vi "Camera.vi"() -> ()   [LabVIEW 2013]
uses:
  Global.vi
panel:
  in  "stop":bool
  in  "Tab Control":enum32{"Camera", "Settings"}(tab)=enum."Settings"
  in  "Pause":bool
  out "Image":T1(plugin-control)
  in  "Zoom":bool
  out "image":i32=1
  in  "max":i32=35000
  in  "min":i32=-35000
  out "Saving":bool=TRUE
  in  "Exposure (ms)":i32=1000
  in  "Colour":u32(ring) items=["Grayscale", "Binary", "Gradient", "Rainbow", "Temperature", "User Defined"]
  out "Image Pixels (I16)":i16[][](array[numeric])=[[-16415, 18069, 30328, 20956, -23719, 10482, 28186, -29010], [32361, 12219, 10367, -21635, -896, 25505, 19841, -22848], [6729, -31829, 19463, -4149, -20618, -4209, 13041, -16224], [-17471, 350, -7557, -30697, 2278, 13038, -13103, -35], [3415, -32273, -5585, -1036, 17798, -25055, 1491, 1884], [10011, -30652, 18549, 30390, 28432, 1602, 13207, 32079], [-19764, -14787, -1537, 876, -26796, 32102, -30010, 10632], [24360, 23280, -15147, -24738, 4016, -28871, -32567, -30048]]
  out "error out":errorcluster
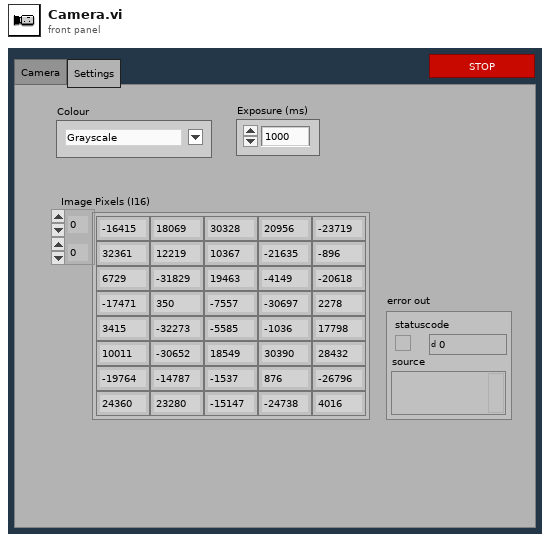
[diagram p1: front panel]
types:
  T1 = typedef "IMAQ Image.ctl" = refnum<image>
  T2 = typedef "Image Type" = u32
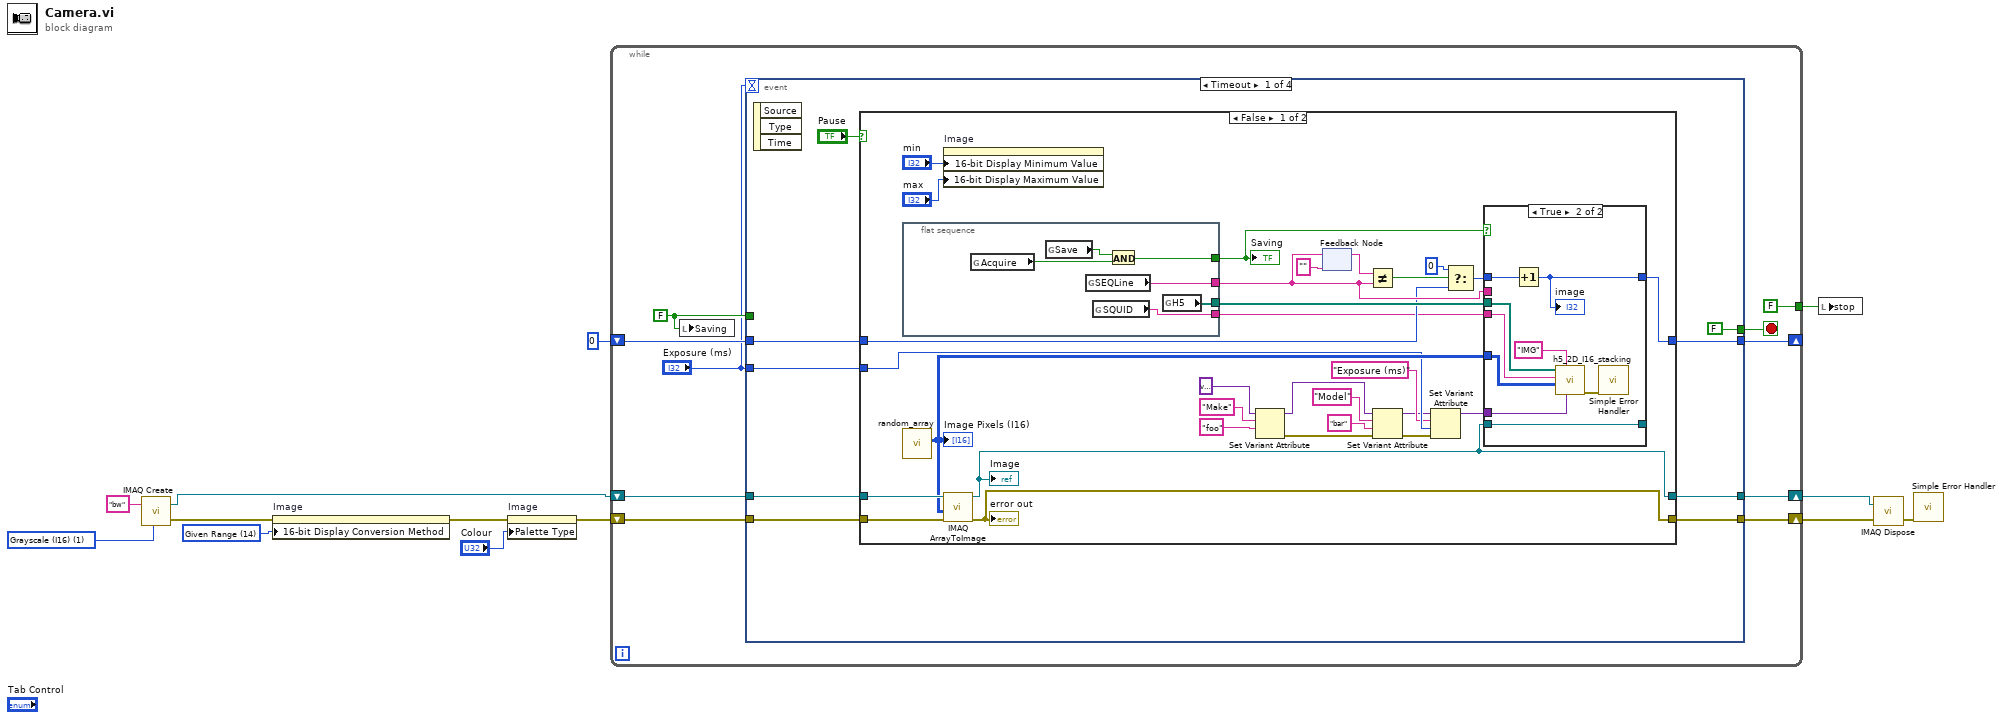
[diagram p0: block diagram]
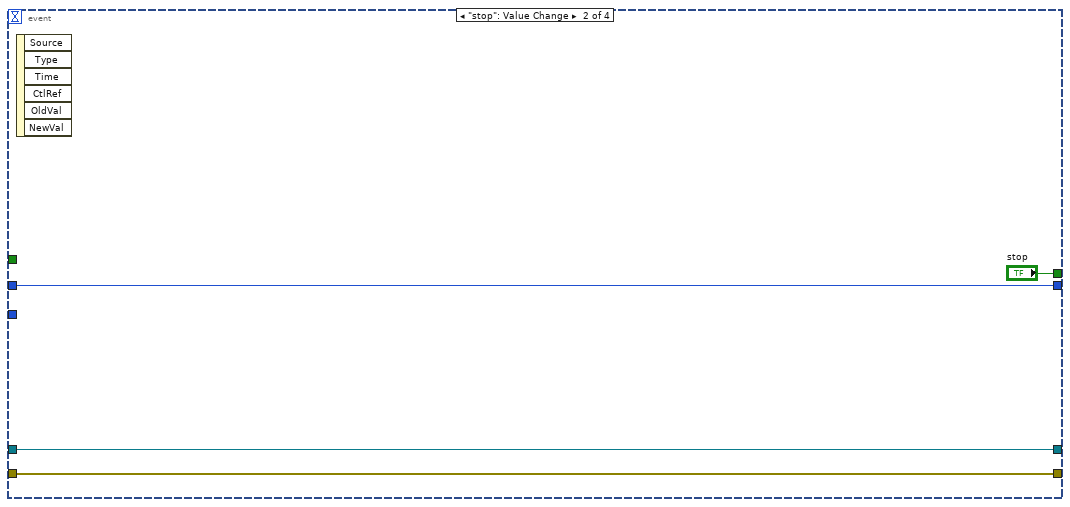
[diagram p4: hidden frame]
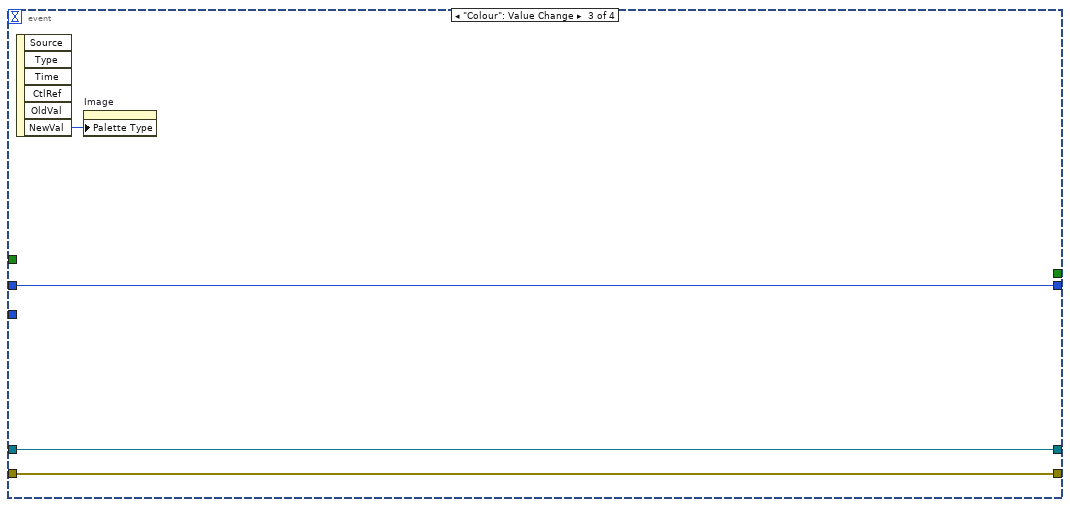
[diagram p5: hidden frame]
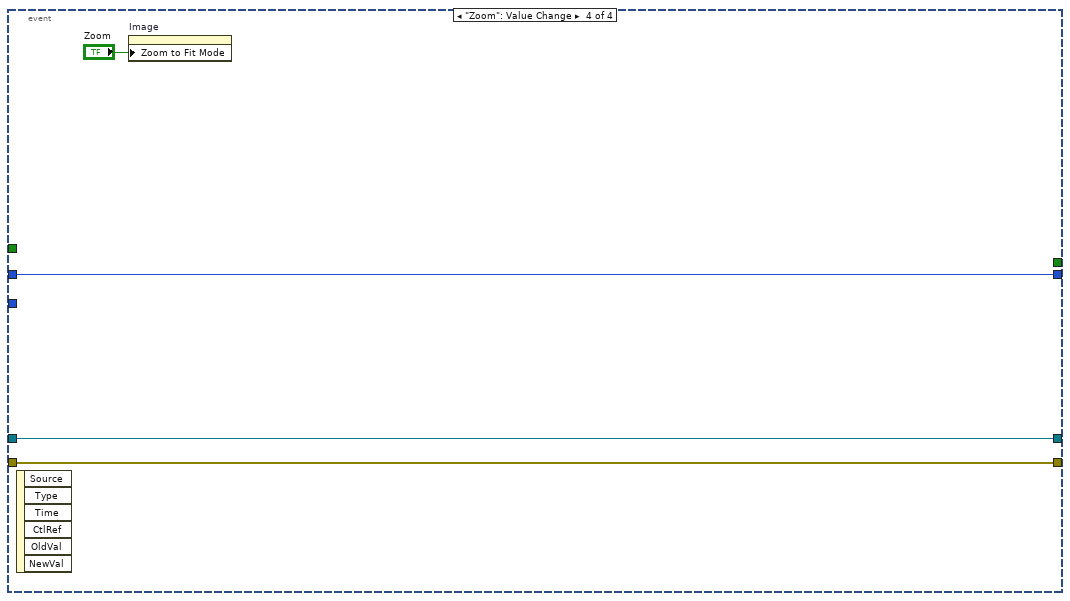
[diagram p6: hidden frame]
diagram:
  w11 = u32 14 items=["Default"=10, "Most Significant Bits"=11, "Full Dynamic"=12, "Downshift"=13, "Given Range"=14, "90% Dynamic"=15, "Given Percent Range"=16] ("16-bit Display Mapping:Conversion Method")
  w13 = T2 1 items=["Grayscale (U8)", "Grayscale (I16)", "Grayscale (SGL)", "Complex (CSG)", "RGB (U32)", "HSL (U32)", "RGB (U64)", "Grayscale (U16)"] ("Image Type")
  n1 = call "IMAQ Create"("Image Name"="bw", "Image Type"=w13) -> ("New Image"=w4:T1, "error out"=w3:errorcluster)  [unwired: 3 in]
  n2 = property on="Image" class="ImageControl"(error in=w3, "16-bit Display Conversion Method"=w11) -> (error out=w8:errorcluster)  [unwired: 1 in, 1 out]
  n3 = property on="Image" class="ImageControl"(error in=w8, "Palette Type"="Colour") -> (error out=w2:errorcluster)  [unwired: 1 in, 1 out]
  n4 = while {
    shift-right: [w23] -> w5
    shift-left: w4 -> [w21]
    shift-right: [w20] -> w1
    shift-left: w2 -> [w19]
    shift-right: [w17] -> _
    shift-left: 0 ("Timeout (ms) 2") -> [w18]
    tunnel: [FALSE ("stop")] -> w6
    stop <- w22 stop-if-true
    w15 = FALSE ("Saving")
    n5 = local write "Saving"(w15) -> ()
    n6 = event shown="[0] Timeout" {
      selector: _ -> [_ _ _ _]
      dyn-events: _ -> [_ _ _ _]
      timeout: "Exposure (ms)" -> [_ _ _ _]
      tunnel: w21 -> [w32 w85 w88 w93]
      tunnel: [w30 w85 w88 w93] -> w23
      tunnel: [FALSE ("Stop") "stop" _ _] -> w22
      tunnel: [w29 w86 w89 w92] -> w20
      tunnel: w19 -> [w31 w86 w89 w92]
      tunnel: w18 -> [w28 w84 w87 w91]
      tunnel: [w27 w84 w87 w91] -> w17
      tunnel: w15 -> [_ _ _ _]
      tunnel: "Exposure (ms)" -> [w24 _ _ _]
      event Timeout {
        n7 = event-data() -> ()  [unwired: 1 in, 3 out]
        n8 = case shown="False" "Pause" {
          tunnel: w32 -> [w50 w82]
          tunnel: w31 -> [w51 w81]
          tunnel: [w49 w82] -> w30
          tunnel: [w48 w81] -> w29
          tunnel: w28 -> [w55 w80]
          tunnel: [w62 w80] -> w27
          tunnel: w24 -> [w37 _]
          frame False {
            n9 = flat-sequence {
              tunnel: [w68] -> w59
              tunnel: [w66] -> w57
              tunnel: [w67] -> w58
              tunnel: [w65] -> w52
              frame #0 {
                n10 = global read "Global.vi" "Acquire"() -> (w63:bool)
                n11 = global read "Global.vi" "Save"() -> (w64:bool)
                n12 = global read "Global.vi" "SEQLine"() -> (w66:string)
                n13 = global read "Global.vi" "SQUID"() -> (w65:string)
                n14 = And(x=w64, y=w63) -> (x .and. y?=w68:bool)
                n15 = global read "Global.vi" "H5"() -> (w67:path[])
              }
            }
            n16 = call "random_array.vi"() -> ("array"=w45:i16[][])  [unwired: 11 in]
            "Image Pixels (I16)" <- w45
            n17 = property on="Image" class="ImageControl"("16-bit Display Minimum Value"="min", "16-bit Display Maximum Value"="max") -> ()  [unwired: 2 in, 2 out]
            n18 = call "IMAQ ArrayToImage"("error in (no error)"=w51, "Image Pixels (I16)"=w45, "Image"=w50) -> ("error out"=w48:errorcluster, "Image Out"=w49:T1)  [unwired: 7 in]
            "Image" <- w49
            "error out" <- w48
            n19 = Set Variant Attribute(Variant=variant ("variant"), name="Make", value="foo" ("Make")) -> (Variant out=w42:variant, error out=w43:errorcluster)  [unwired: 1 in, 1 out]
            n20 = feedback #1("" ("Seq")) -> (w60:string)
            n21 = feedback-in #1(w57) -> ()
            n22 = Not Equal?(x=w60, y=w57) -> (x != y?=w53:bool)
            n23 = Set Variant Attribute(Variant=w42, name="Model", value="bar" ("name"), error in=w43) -> (Variant out=w34:variant, error out=w35:errorcluster)  [unwired: 1 out]
            n24 = Set Variant Attribute(Variant=w34, name="Exposure (ms)", value=w37, error in=w35) -> (Variant out=w33:variant)  [unwired: 2 out]
            n25 = Select(t=0 ("Timeout (ms) 2"), s=w53, f=w55) -> (s? t:f=w56:i32)
            n26 = case shown="True" w59 {
              tunnel: [w70 w77] -> _
              tunnel: w49 -> [w70 w77]
              tunnel: w56 -> [w69 w79]
              tunnel: [w69 w78] -> w62
              tunnel: w58 -> [_ w76]
              tunnel: w57 -> [_ _]
              tunnel: w52 -> [_ w74]
              tunnel: w45 -> [_ w72]
              tunnel: w33 -> [_ w71]
              frame False {
              }
              frame True {
                n27 = Increment(x=w79) -> (x+1=w78:i32)
                "image" <- w78
                n28 = call "h5_2D_I16_stacking.vi"("Attributes"=w71, "TYPE"="IMG", "2D I16"=w72, "SQUID"=w74, "H5"=w76) -> ("error out"=w73:errorcluster)  [unwired: 5 in, 1 out]
                n29 = call <vilib>:"Simple Error Handler.vi"("error in (no error)"=w73) -> ()  [unwired: 4 in, 5 out]
              }
            }
            "Saving" <- w59
          }
          frame True {
          }
        }
      }
      event "stop": Value Change {
        n30 = event-data() -> ()  [unwired: 1 in, 6 out]
      }
      event "Colour": Value Change {
        n31 = event-data() -> ("NewVal"=w90:u32)  [unwired: 1 in, 5 out]
        n32 = property on="Image" class="ImageControl"("Palette Type"=w90) -> ()  [unwired: 2 in, 2 out]
      }
      event "Zoom": Value Change {
        n33 = event-data() -> ()  [unwired: 1 in, 6 out]
        n34 = property on="Image" class="ImageControl"("Zoom to Fit Mode"="Zoom") -> ()  [unwired: 2 in, 2 out]
      }
    }
  }
  n35 = local write "stop"(w6) -> ()
  n36 = call "IMAQ Dispose"("Image"=w5, "error in (no error)"=w1) -> ("error out"=w10:errorcluster)  [unwired: 4 in]
  n37 = call <vilib>:"Simple Error Handler.vi"("error in (no error)"=w10) -> ()  [unwired: 4 in, 5 out]
